vi "OpenCVFaceDetection_SendUiEvent.vi"(7 "UiEventNames":T1, 8 "ErrorIn":errorcluster, 9 "Data":variant, 11 "OpenCVFaceDetectionIn":refnum<class "OpenCVFaceDetection.lvclass">) -> (0 "ErrorOut":errorcluster, 3 "OpenCVFaceDetectionOut":refnum<class "OpenCVFaceDetection.lvclass">)   [LabVIEW 2021, in "OpenCVFaceDetection.lvclass"]
doc: "Sends the selected event to the registered event handler loops in the user interface VI."
uses:
  OpenCVFaceDetection.lvclass
  OpenCVFaceDetection_UiCallBackEvents.ctl
  OpenCVFaceDetection.lvclass/OpenCVFaceDetection.ctl
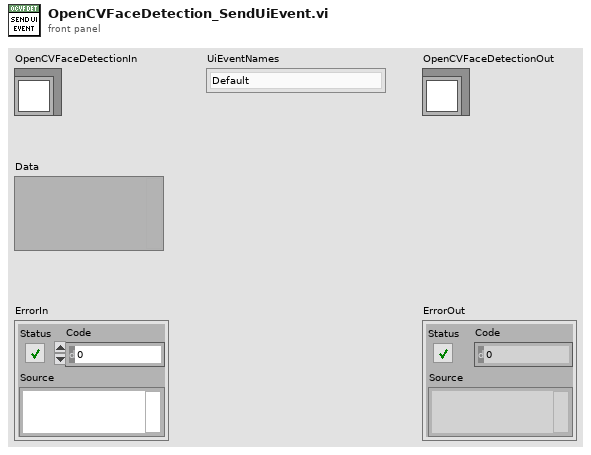
[diagram p1: front panel]
types:
  T1 = typedef "OpenCVFaceDetection.lvclass/OpenCVFaceDetection_UiCallBackEvents.ctl" = enum16{"Default", "PersistentDataUpdated", "NewPicture", "Worker 1: Do Something"}
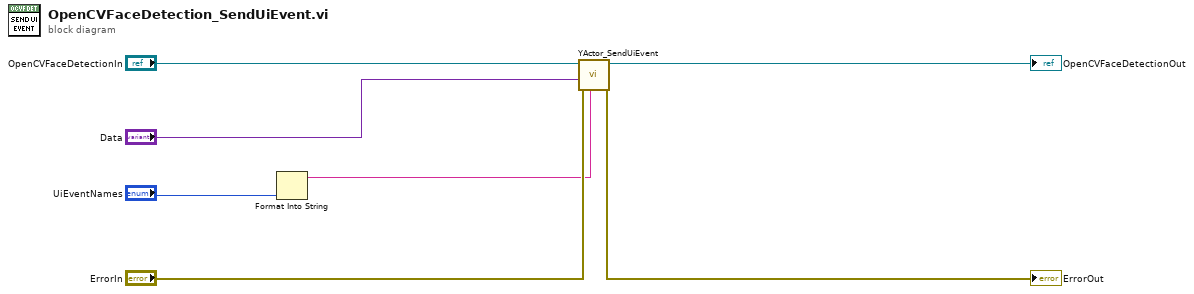
[diagram p0: block diagram]
diagram:
  n1 = Format Into String("UiEventNames") -> (resulting string=w2:string)  [unwired: 3 in, 1 out]
  n2 = call-dynamic "YActor_SendUiEvent.vi"("Event"=w2, "ErrorIn"="ErrorIn", "Data"="Data", "YActorIn"="OpenCVFaceDetectionIn") -> ("ErrorOut"=→"ErrorOut":errorcluster, "YActorOut"=→"OpenCVFaceDetectionOut":refnum<class "OpenCVFaceDetection.lvclass">)  [unwired: 6 in]
